vi "Tool measurment data collection.vi"(1 "Quer loop":u16, 2 "Stat 2 reader ID":i32, 11 "error out":errorcluster) -> ()   [LabVIEW 2011]
uses:
  LEINmaster/Defenitions/LEIN Structure variations.ctl
  LEINmaster/Defenitions/LEIN CMD List.ctl
  Stroker/Stat def/Stroker system stat2.ctl
  LEINmaster/Nodes/Controller local stat2.ctl
  LEINmaster/Nodes/pressure stat2.ctl
  LEINmaster/Nodes/solonoid stat2.ctl
  LEINmaster/Nodes/PSU stat2.ctl
  LEINmaster/Nodes/tensionsub stat2.ctl
  LEINmaster/Nodes/STAT2 data carrier type aware.ctl
  List of tools.ctl
  emi Lib/System 01/0 - General/App/Loop control 2/Private/_emi_ SMLoop start condition.vi
  emi Lib/System 01/0 - General/App/Loop control 2/Private/_emi_ SMLoop Error Check.vi
  emi Lib/Basic/0 - General/Error/emi_Is Error.vi
  emi Lib/System 01/0 - General/App/Loop control 2/Private/_emi_SMLoop Register new.vi
  emi Lib/System 01/0 - General/S&E reporting/emi_Send S&E Error message.vi
  emi Lib/Basic/0 - General/Error/emi_ Is Error state.vi
  emi Lib/System 01/0 - General/emi_Read System ID.vi
  emi Lib/System 01/0 - General/App/Loop control/Private/_emi_GFV Loop Linking.vi
  emi Lib/System 01/0 - General/App/Loop control/Private/_emi_GFV Loop Enable.vi
  emi Lib/System 01/0 - General/App/Loop control 2/Private/_emi_ SMLoop Restart.vi
  emi Lib/System 01/0 - General/App/Private/_emi_GFV App Close.vi
  emi Lib/System 01/0 - General/App/Loop control 2/Private/_emi_ SMLoop Restart Counter.vi
  emi Lib/System 01/0 - General/App/Loop control/Private/_emi_GFV Loop Running.vi
  emi Lib/System 01/0 - General/Private/_emi_GFV System ID.vi
  emi Lib/System 01/0 - General/S&E reporting/Private/_emi_S&E Q Generator.vi
  <vilib>/Utility/error.llb/Clear Errors.vi
  emi Lib/System 01/0 - General/App/Loop control/Private/_emi_GFV stop a loop so it can reset.vi
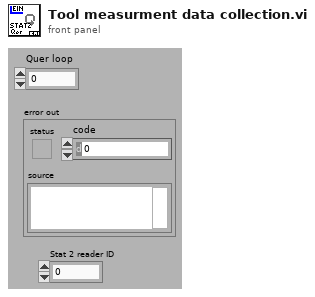
[diagram p1: front panel]
types:
  T1 = typedef "LEIN custom reply Q.ctl" = refnum<queue>
  T2 = typedef "LEIN CMD List.ctl" = enum8{"ACTI", "TASK", "RES0", "STAT", "RES1", "RES2", "RES3", "USER"}
  T3 = typedef "Stroker system stat2.ctl" = cluster{"Controller local":T4, "pressure 1":T5, "pressure 2":T5, "solonoid":T6, "PSU":T7, "Tension Sub 1":T8, "Tension Sub 2":T8}
  T4 = typedef "Controller local stat2.ctl" = cluster{"sys register":u16, "temperature":u16, "Input voltage":u16, "Input Current":u16, "Accelerometer ch0":u16, "Accelerometer ch1":u16, "Accelerometer ch2":u16, "Relay status":u8, "GPIO values":u8, "Sensor 1":i32, "Sensor 2":i32, "NA":u8, "High G monitoring":u8}
  T5 = typedef "pressure stat2.ctl" = cluster{"sys register":u16, "temperature":u16, "Pressure":u16, "osctun":u8}
  T6 = typedef "solonoid stat2.ctl" = cluster{"sys register":u16, "temperature":u16, "Position":i16, "monitor state":u8, "valve status":u8}
  T7 = typedef "PSU stat2.ctl" = cluster{"sys register":u16, "temperature":u16, "HV Voltage in":u16, "Main Voltage out":u16, "Main Current out":u16}
  T8 = typedef "tensionsub stat2.ctl" = cluster{"sys register":u16, "temperature":u16, "Tension":i16, "osctun":u8}
  T9 = typedef "STAT2 data carrier type aware.ctl" = cluster{"Tool":T10, "Data":variant}
  T10 = typedef "List of tools.ctl" = enum16{"Stroker", "Driller", "Tractor"}
  T11 = enum16{"big-endian, network order", "native, host order", "little-endian"}
  T12 = typedef "_emi_ SMLoop sates.ctl" = enum16{"Init", "Standby", "Start", "Normal Operation", "Stop", "Error Handling", "End", "Post"}
  T13 = cluster{"Placeholder":bool, "time valid receive":i32}
  T14 = typedef "LEIN Reply Holder.ctl" = cluster{"Reply msg(cmdif no reply)":T15, "Reply time":timestamp, "Valid reply":bool}
  T15 = typedef "LEIN CMD Cluster.ctl" = cluster{"SID":u8, "ANF":bool, "CMD":T2, "DATA":u8[]}
  T16 = typedef "LEIN Structure variations.ctl" = enum16{"LEIN08", "LEIN31", "LEIN63"}
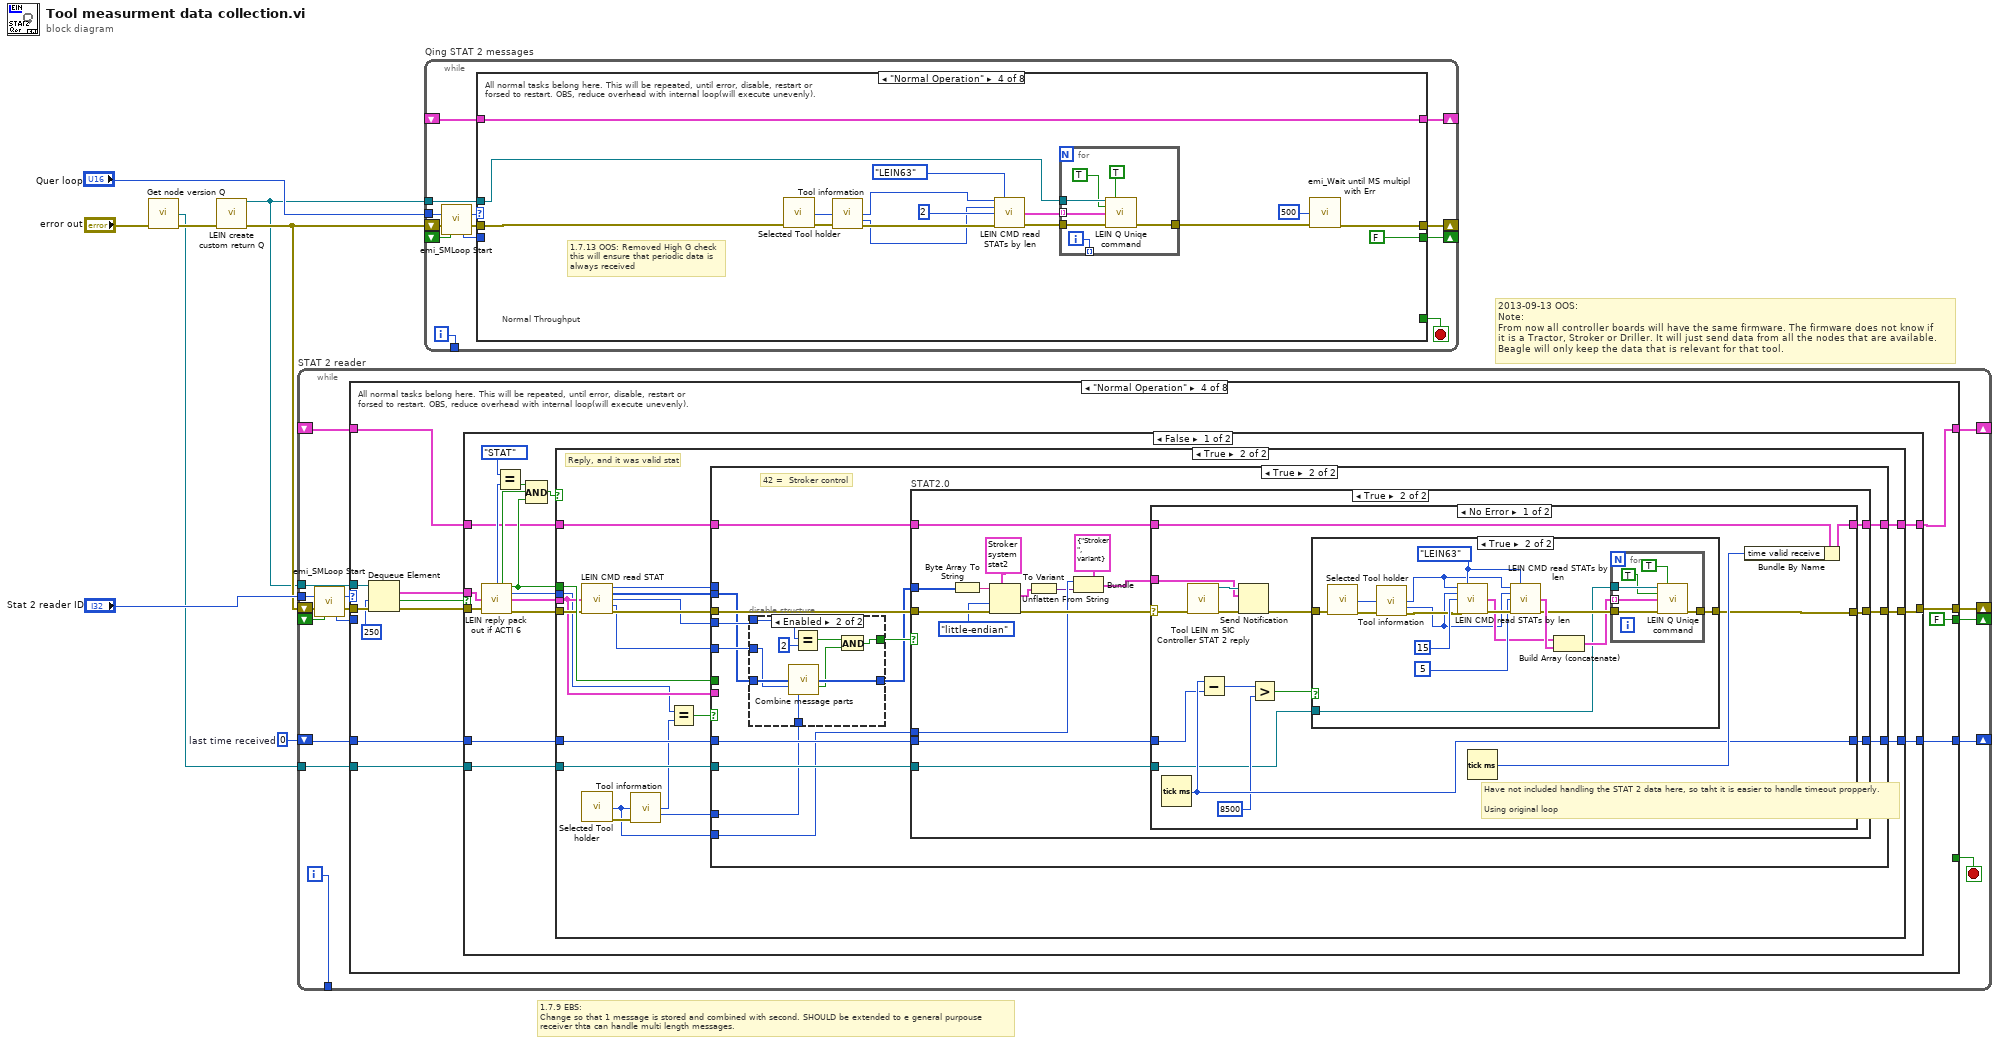
[diagram p0: block diagram]
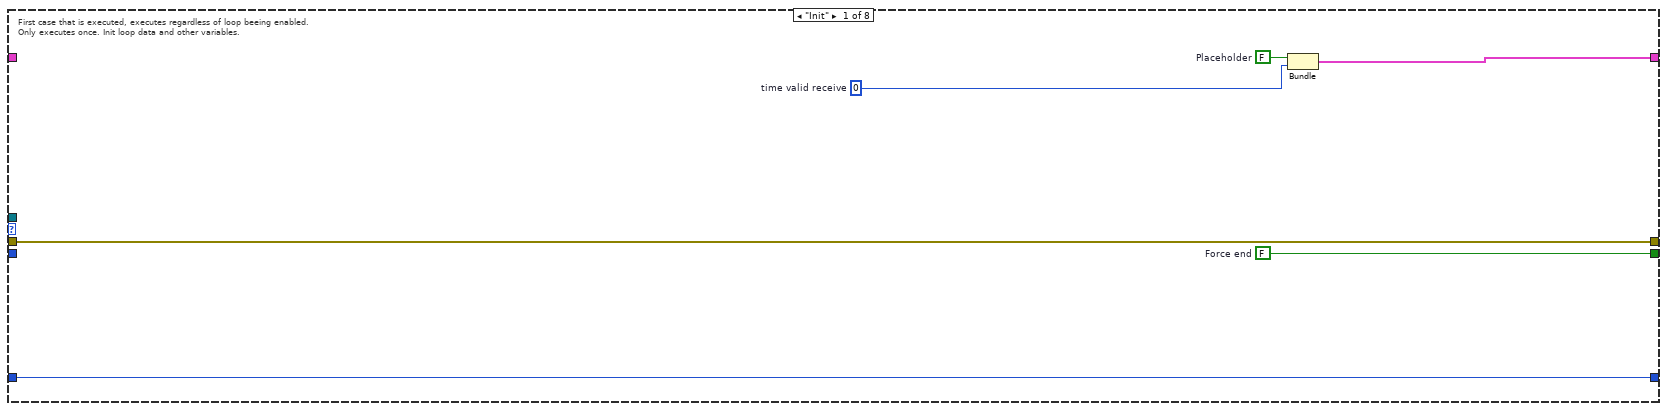
[diagram p2: hidden frame]
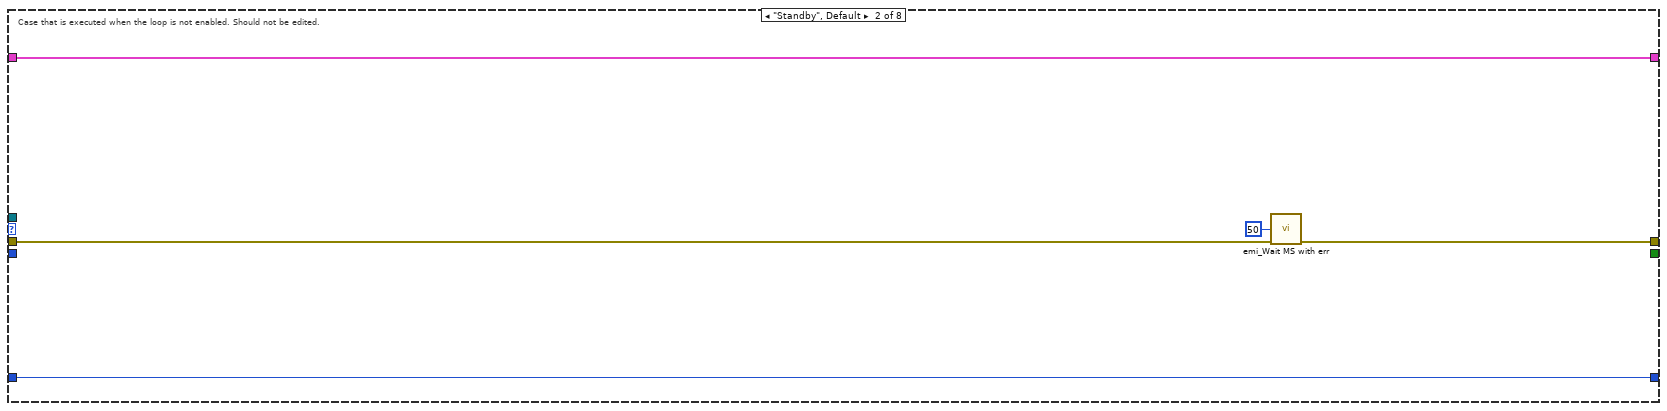
[diagram p3: hidden frame]
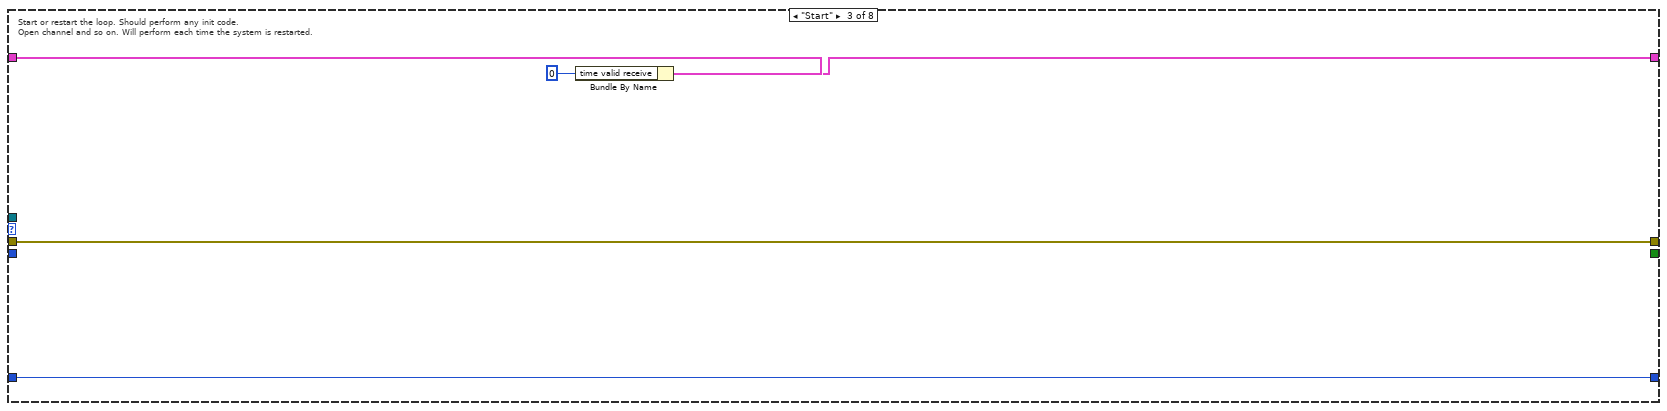
[diagram p4: hidden frame]
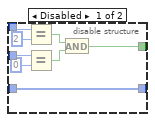
[diagram p7: hidden frame]
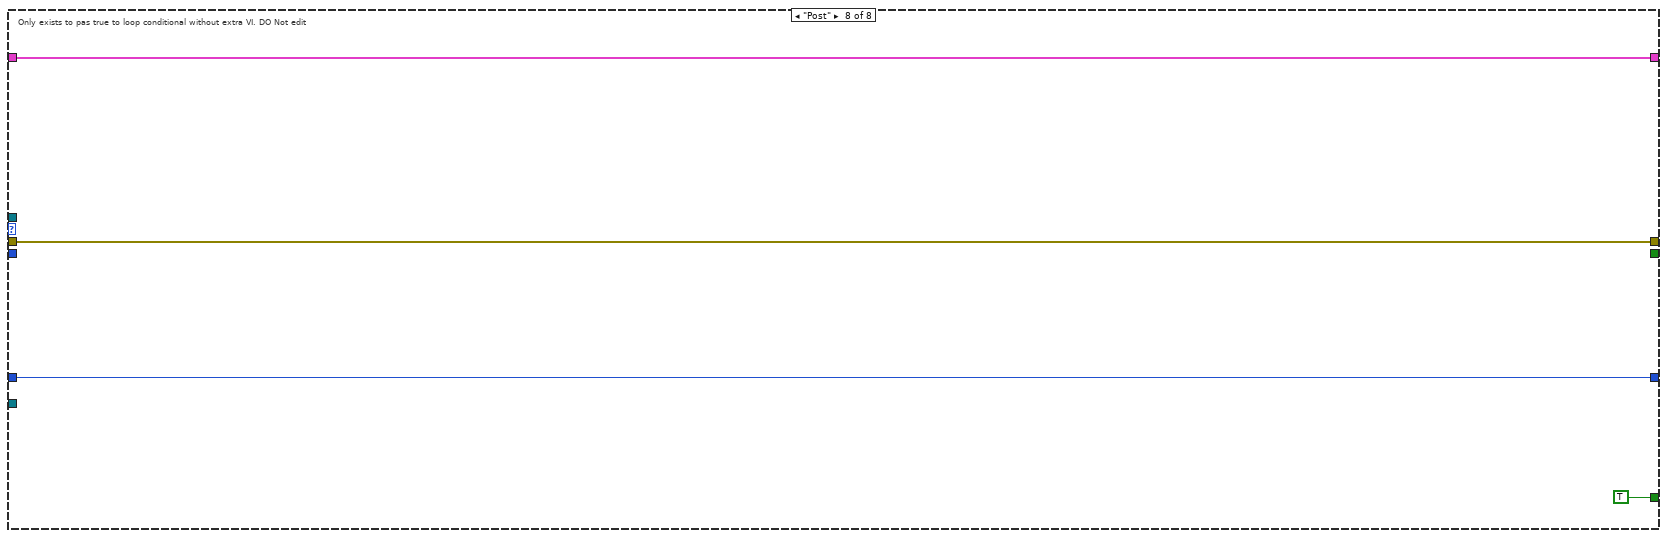
[diagram p15: hidden frame]
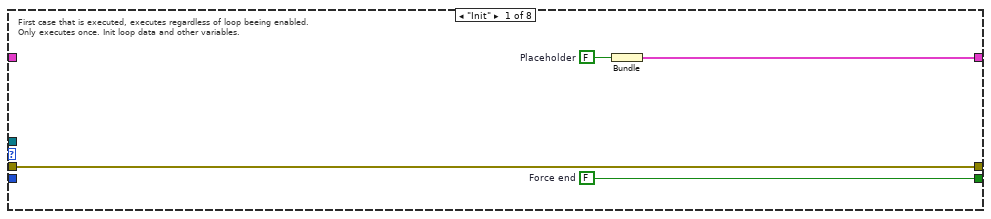
[diagram p16: hidden frame]
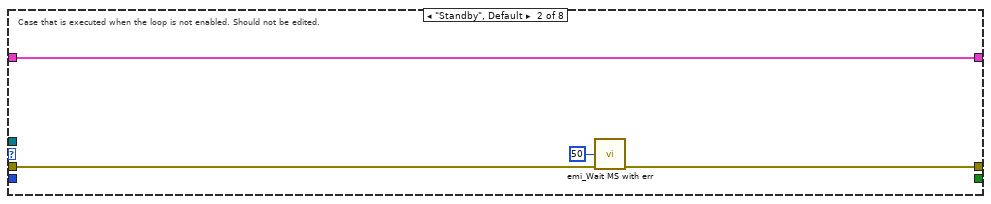
[diagram p17: hidden frame]
diagram:
  w4 = u32 0  # last time received
  # "2013-09-13 OOS:\nNote: \nFrom now all controller boards will have the same firmware. The firmware does not know if\nit is a Tractor, Stroker or Driller. It will just send data from all the nodes that are available. \nBeagle will only keep the data that is relevant for that tool."
  # "1.7.9 EBS:\nChange so that 1 message is stored and combined with second. SHOULD be extended to e general purpouse \nreceiver thta can handle multi length messages."
  n1 = call "Get node version Q.vi"("error in"="error out") -> ("LEIN custom reply Q"=w1:T1, "error out"=w2:errorcluster)  [unwired: 13 in]
  n2 = call "LEIN create custom return Q.vi"("error in (no error)"=w2) -> ("LEIN custom reply Q"=w5:T1, "error out"=w6:errorcluster)  [unwired: 13 in]
  n3 = while "STAT 2 reader" {
    shift-right: [w24] -> _
    shift-left: _ -> [w20]
    shift-right: [w22] -> _
    shift-left: w6 -> [w18]
    tunnel: [w21] -> _
    shift-right: [w19] -> _
    shift-left: _ -> [w14]
    tunnel: "Stat 2 reader ID" -> [w15]
    tunnel: w5 -> [w12]
    shift-right: [w11] -> _
    shift-left: w4 -> [w10]
    tunnel: w1 -> [w9]
    i -> [w21]
    stop <- w23 stop-if-true
    n4 = call "emi_SMLoop Start.vi"("Loop ID"=w15, "error in (no error)"=w18, "Force Stop(F)"=w14) -> ("Loop command"=w16:T12, "error out"=w17:errorcluster, "Loop ID out"=w13:i32)  [unwired: 10 in]
    n5 = case shown="\"Normal Operation\"" w16 {
      tunnel: [w29 w32 w38 w44 w193 w197 w199 w203] -> w24
      tunnel: [_ _ _ _ _ _ _ TRUE] -> w23
      tunnel: w17 -> [w30 w34 w40 w52 w194 w196 w200 w204]
      tunnel: [w30 w33 w40 w47 w194 w196 w200 w204] -> w22
      tunnel: w20 -> [_ w32 w39 w45 w193 w197 w199 w203]
      tunnel: [w27 _ _ FALSE ("Force End") _ _ _ _] -> w19
      tunnel: w13 -> [_ _ _ _ _ _ _ _]
      tunnel: w12 -> [_ _ _ w51 _ _ _ _]
      tunnel: [w25 w31 w36 w43 w192 w195 w198 w201] -> w11
      tunnel: w10 -> [w25 w31 w36 w42 w192 w195 w198 w201]
      tunnel: w9 -> [_ _ _ w41 _ _ _ _]
      frame "Init" {
        w26 = 0  # time valid receive
        w27 = FALSE  # Force end
        w28 = FALSE  # Placeholder
        # "First case that is executed, executes regardless of loop beeing enabled.\nOnly executes once. Init loop data and other variables."
        n6 = Bundle("Placeholder"=w28, "time valid receive"=w26) -> (w29:T13)  [unwired: 1 in]
      }
      frame "Standby", Default {
        # "Case that is executed when the loop is not enabled. Should not be edited."
        n7 = call "emi_Wait MS with err.vi"("milliseconds to wait(0)"=u32 50, "error in (no error)"=w34) -> ("error out"=w33:errorcluster)  [unwired: 13 in]
      }
      frame "Start" {
        # "Start or restart the loop. Should perform any init code. \nOpen channel and so on. Will perform each time the system is restarted."
        n8 = Bundle By Name(cluster=w39, "time valid receive"=0) -> (w38:T13)
      }
      frame "Normal Operation" {
        # "All normal tasks belong here. This will be repeated, until error, disable, restart or\nforsed to restart. OBS, reduce overhead with internal loop(will execute unevenly)."
        n9 = Dequeue Element(queue=w51, timeout in ms (-1)=250, error in (no error)=w52) -> (element=w46:T14, timed out?=w49:bool, error out=w48:errorcluster)  [unwired: 1 out]
        n10 = case shown="False" w49 {
          tunnel: w48 -> [w70 w190]
          tunnel: [w67 w190] -> w47
          tunnel: w46 -> [w69 _]
          tunnel: w45 -> [w58 w191]
          tunnel: [w57 w191] -> w44
          tunnel: [w56 w189] -> w43
          tunnel: w42 -> [w55 w189]
          tunnel: w41 -> [w54 _]
          frame False {
            n11 = call "LEIN reply pack out if ACTI 6.vi"("LEIN reply holder"=w69, "error in (no error)"=w70) -> ("CMD"=w61:T2, "Valid reply"=w64:bool, "ANF"=w62:bool, "SID"=w65:u8, "Reply(CMD if no reply)"=w66:T15, "error out"=w68:errorcluster)  [unwired: 8 in]
            n12 = Equal?(x=LEIN_CMD_List."STAT", y=w61) -> (x = y?=w59:bool)
            n13 = Compound Arithmetic op=AND(w59, w64, w62) -> (w63:bool)
            n14 = case shown="True" w63 {
              tunnel: w68 -> [w73 w91]
              tunnel: [w73 w93] -> w67
              tunnel: w66 -> [_ w90]
              tunnel: w65 -> [_ w78]
              tunnel: w62 -> [_ w92]
              tunnel: w58 -> [w72 w84]
              tunnel: [w72 w83] -> w57
              tunnel: [w71 w82] -> w56
              tunnel: w55 -> [w71 w81]
              tunnel: w54 -> [_ w80]
              frame False {
                # "No reply, or a NACK reply."
              }
              frame True {
                # "Reply, and it was valid stat"
                n15 = call "LEIN CMD read STAT.vi"("CMD"=w90, "error in (no error)"=w91) -> ("SID"=w86:u8, "Data"=w88:u8[], "STAT ID"=w87:u8, "STAT Part"=w85:u8, "error out"=w89:errorcluster)  [unwired: 8 in, 1 out]
                n16 = call "Selected Tool holder.vi"() -> ("Tool out"=w75:T10, "error out"=w76:errorcluster)  [unwired: 14 in]
                n17 = call "Tool information.vi"("Tool in"=w75, "error in (no error)"=w76) -> ("Main node address"=w79:u8, "Expected stat 2 message len"=w74:u8)  [unwired: 10 in, 2 out]
                n18 = Equal?(x=w78, y=w79) -> (x = y?=w77:bool)
                n19 = case shown="True" w77 {
                  tunnel: [w96 w107] -> w93
                  tunnel: w89 -> [w96 w106]
                  tunnel: w90 -> [_ _]
                  tunnel: w92 -> [_ _]
                  tunnel: w88 -> [_ w100]
                  tunnel: w87 -> [_ w109]
                  tunnel: w86 -> [_ _]
                  tunnel: w85 -> [_ w110]
                  tunnel: w84 -> [w95 w105]
                  tunnel: [w95 w104] -> w83
                  tunnel: [w94 w103] -> w82
                  tunnel: w81 -> [w94 w102]
                  tunnel: w80 -> [_ w101]
                  tunnel: w75 -> [_ w97]
                  tunnel: w74 -> [_ w98]
                  frame False {
                    # "TODO: Error?"
                  }
                  frame True {
                    # "42 =  Stroker control"
                    n20 = disable-structure shown="Enabled" {
                      disable-tunnel: w110 -> [w118 w121]
                      disable-tunnel: w109 -> [w117 w127]
                      disable-tunnel: [w112 w124] -> w108
                      disable-tunnel: w100 -> [w111 w123]
                      disable-tunnel: [w111 w122] -> w99
                      disable-tunnel: w98 -> [_ w119]
                      frame Disabled {
                        n21 = Equal?(x=w117, y=u8 2) -> (x = y?=w114:bool)
                        n22 = Equal?(x=w118, y=u8 0) -> (x = y?=w113:bool)
                        n23 = And(x=w114, y=w113) -> (x .and. y?=w112:bool)
                      }
                      frame Enabled {
                        n24 = call "Combine message parts.vi"("Data"=w123, "part"=w121, "Expected bytes"=w119) -> ("Data complete"=w122:u8[], "Complete data"=w120:bool)  [unwired: 11 in]
                        n25 = Equal?(x=w127, y=u8 2) -> (x = y?=w125:bool)
                        n26 = And(x=w125, y=w120) -> (x .and. y?=w124:bool)
                      }
                    }
                    n27 = case "STAT2.0" shown="True" w108 {
                      tunnel: [w129 w142] -> w107
                      tunnel: w106 -> [w129 w147]
                      tunnel: w99 -> [_ w146]
                      tunnel: w105 -> [w130 w144]
                      tunnel: [w130 w143] -> w104
                      tunnel: [w128 w140] -> w103
                      tunnel: w102 -> [w128 w139]
                      tunnel: w101 -> [_ w138]
                      tunnel: w97 -> [_ w137]
                      frame False {
                      }
                      frame True {
                        n28 = Byte Array To String(unsigned byte array=w146) -> (string=w136:string)
                        n29 = Unflatten From String(type=T3 {"Controller local"={"sys register"=0, "temperature"=0, "Input voltage"=0, "Input Current"=0, "Accelerometer ch0"=0, "Accelerometer ch1"=0, "Accelerometer ch2"=0, "Relay status"=0, "GPIO values"=0, "Sensor 1"=0, "Sensor 2"=0, "NA"=0, "High G monitoring"=0}, "pressure 1"={"sys register"=0, "temperature"=0, "Pressure"=0, "osctun"=0}, "pressure 2"={"sys register"=0, "temperature"=0, "Pressure"=0, "osctun"=0}, "solonoid"={"sys register"=0, "temperature"=0, "Position"=0, "monitor state"=0, "valve status"=0}, "PSU"={"sys register"=0, "temperature"=0, "HV Voltage in"=0, "Main Voltage out"=0, "Main Current out"=0}, "Tension Sub 1"={"sys register"=0, "temperature"=0, "Tension"=0, "osctun"=0}, "Tension Sub 2"={"sys register"=0, "temperature"=0, "Tension"=0, "osctun"=0}} ("system stat2"), binary string=w136, byte order (0:big-endian, network order)=T11."little-endian", error in (no error)=w147) -> (value=w132:T3, error out=w145:errorcluster)  [unwired: 1 in, 1 out]
                        n30 = To Variant(anything=w132) -> (Variant=w131:variant)
                        n31 = Bundle(cluster=T9 {"Tool"=enum."Stroker", "Data"=variant}, "Tool"=w137, "Data"=w131) -> (w141:T9)
                        n32 = case shown="No Error" w145 {
                          selector: w145 -> [w158 w187]
                          tunnel: w144 -> [w162 w188]
                          tunnel: [w161 w188] -> w143
                          tunnel: [w151 w187] -> w142
                          tunnel: w141 -> [w156 _]
                          tunnel: [w155 w186] -> w140
                          tunnel: w139 -> [w154 w186]
                          tunnel: w138 -> [w149 _]
                          frame No Error {
                            # "Have not included handling the STAT 2 data here, so taht it is easier to handle timeout propperly.\n\nUsing original loop"
                            n33 = Tick Count (ms)() -> (millisecond timer value=w155:u32)
                            n34 = call "Tool LEIN m SIC Controller STAT 2 reply.vi"("error in (no error)"=w158) -> ("notifier out"=w159:refnum<notifier>, "error out"=w157:errorcluster)  [unwired: 13 in]
                            n35 = Subtract(x=w155, y=w154) -> (x-y=w153:u32)
                            n36 = Send Notification(notification=w156, notifier=w159, error in (no error)=w157) -> (error out=w148:errorcluster)  [unwired: 1 out]
                            n37 = Greater?(x=w153, y=u32 8500) -> (0:w150:bool)
                            n38 = case shown="True" w150 {
                              tunnel: [w163 w173] -> w151
                              tunnel: w148 -> [w163 w164]
                              tunnel: w149 -> [_ w170]
                              frame False {
                              }
                              frame True {
                                w176 = LEIN_Structure_variations."LEIN63" ("LEIN Variation")
                                n39 = call "Selected Tool holder.vi"("error in (no error)"=w164) -> ("Tool out"=w168:T10, "error out"=w169:errorcluster)  [unwired: 13 in]
                                n40 = call "Tool information.vi"("Tool in"=w168, "error in (no error)"=w169) -> ("Main node address"=w166:u8, "Expected stat 2 message len"=w165:u8, "error out"=w167:errorcluster)  [unwired: 10 in, 1 out]
                                n41 = call "LEIN CMD read STATs by len.vi"("SID"=w166, "LEIN Variation"=w176, "Expected LEN"=w165, "STAT ID"=u8 15, "error in"=w167) -> ("STATs"=w174:T15[], "error out"=w178:errorcluster)  [unwired: 9 in]
                                n42 = call "LEIN CMD read STATs by len.vi"("SID"=w166, "LEIN Variation"=w176, "Expected LEN"=w165, "STAT ID"=u8 5, "error in"=w178) -> ("STATs"=w175:T15[], "error out"=w172:errorcluster)  [unwired: 9 in]
                                n43 = Build Array (concatenate)(w174, w175) -> (w171:T15[])
                                n44 = for {
                                tunnel: [w185] -> w173
                                tunnel: w172 -> [w184]
                                tunnel: w171 -> [w183] mode=indexing
                                tunnel: w170 -> [w181]
                                n45 = call "LEIN Q Uniqe command.vi"("LEIN custom reply Q"=w181, "Retry on err (F)"=TRUE, "Custom Q(F)"=TRUE, "CMD"=w183, "error in"=w184) -> ("error out"=w185:errorcluster)  [unwired: 10 in]
                                }
                              }
                            }
                            n46 = Tick Count (ms)() -> (millisecond timer value=w160:u32)
                            n47 = Bundle By Name(cluster=w162, "time valid receive"=w160) -> (w161:T13)
                          }
                          frame Error {
                          }
                        }
                      }
                    }
                  }
                }
              }
            }
          }
          frame True {
          }
        }
      }
      frame "Stop" {
        # "Stop the loop. May be restarted later. Close interfaces and the like"
      }
      frame "Error Handling" {
        # "Loop automaticaly returns here after error is found. If error is cleared, \nLoop wil continue as normal(if was operative when error."
      }
      frame "End" {
        # "Only executes at application end has. Should performa any action the loop \nneeds to finnish. Executes only once."
      }
      frame "Post" {
        # "Only exists to pas true to loop conditional without extra VI. DO Not edit"
      }
    }
  }
  n48 = while "Qing STAT 2 messages" {
    shift-right: [w217] -> _
    shift-left: _ -> [w213]
    shift-right: [w215] -> _
    shift-left: w6 -> [w211]
    tunnel: [w214] -> _
    shift-right: [w212] -> _
    shift-left: _ -> [w207]
    tunnel: "Quer loop" -> [w208]
    tunnel: w5 -> [w205]
    i -> [w214]
    stop <- w216 stop-if-true
    n49 = call "emi_SMLoop Start.vi"("Loop ID"=w208, "error in (no error)"=w211, "Force Stop(F)"=w207) -> ("Loop command"=w209:T12, "error out"=w210:errorcluster, "Loop ID out"=w206:i32)  [unwired: 10 in]
    n50 = case shown="\"Normal Operation\"" w209 {
      tunnel: [w220 w222 w226 w241 w251 w254 w255 w258] -> w217
      tunnel: [_ _ _ _ _ _ _ TRUE] -> w216
      tunnel: w210 -> [w221 w224 w227 w243 w252 w253 w256 w259]
      tunnel: [w221 w223 w227 w242 w252 w253 w256 w259] -> w215
      tunnel: w213 -> [_ w222 w226 w241 w251 w254 w255 w258]
      tunnel: [w218 _ _ FALSE ("Force End") _ _ _ _] -> w212
      tunnel: w206 -> [_ _ _ _ _ _ _ _]
      tunnel: w205 -> [_ _ _ w239 _ _ _ _]
      frame "Init" {
        w218 = FALSE  # Force end
        w219 = FALSE  # Placeholder
        # "First case that is executed, executes regardless of loop beeing enabled.\nOnly executes once. Init loop data and other variables."
        n51 = Bundle("Placeholder"=w219) -> (w220:cluster{"Placeholder":bool})  [unwired: 1 in]
      }
      frame "Standby", Default {
        # "Case that is executed when the loop is not enabled. Should not be edited."
        n52 = call "emi_Wait MS with err.vi"("milliseconds to wait(0)"=u32 50, "error in (no error)"=w224) -> ("error out"=w223:errorcluster)  [unwired: 13 in]
      }
      frame "Start" {
        # "Start or restart the loop. Should perform any init code. \nOpen channel and so on. Will perform each time the system is restarted."
      }
      frame "Normal Operation" {
        # "1.7.13 OOS: Removed High G check\nthis will ensure that periodic data is \nalways received"
        # "Normal Throughput"
        # "All normal tasks belong here. This will be repeated, until error, disable, restart or\nforsed to restart. OBS, reduce overhead with internal loop(will execute unevenly)."
        n53 = call "Selected Tool holder.vi"("error in (no error)"=w243) -> ("Tool out"=w231:T10, "error out"=w232:errorcluster)  [unwired: 13 in]
        n54 = call "Tool information.vi"("Tool in"=w231, "error in (no error)"=w232) -> ("Main node address"=w230:u8, "Expected stat 2 message len"=w228:u8, "error out"=w229:errorcluster)  [unwired: 10 in, 1 out]
        n55 = call "LEIN CMD read STATs by len.vi"("SID"=w230, "LEIN Variation"=LEIN_Structure_variations."LEIN63", "Expected LEN"=w228, "STAT ID"=u8 2, "error in"=w229) -> ("STATs"=w234:T15[], "error out"=w235:errorcluster)  [unwired: 9 in]
        n56 = for {
          tunnel: [w250] -> w237
          tunnel: w235 -> [w249]
          tunnel: w234 -> [w248] mode=indexing
          tunnel: w239 -> [w246]
          tunnel: [w244] -> _ mode=indexing
          i -> [w244]
          n57 = call "LEIN Q Uniqe command.vi"("LEIN custom reply Q"=w246, "Retry on err (F)"=TRUE, "Custom Q(F)"=TRUE, "CMD"=w248, "error in"=w249) -> ("error out"=w250:errorcluster)  [unwired: 10 in]
        }
        n58 = call "emi_Wait until MS multipl with Err.vi"("millisecond multiple(0)"=u32 500 ("milliseconds to wait(0)"), "error in (no error)"=w237) -> ("error out"=w242:errorcluster)  [unwired: 13 in]
      }
      frame "Stop" {
        # "Stop the loop. May be restarted later. Close interfaces and the like"
      }
      frame "Error Handling" {
        # "Loop automaticaly returns here after error is found. If error is cleared, \nLoop wil continue as normal(if was operative when error."
      }
      frame "End" {
        # "Only executes at application end has. Should performa any action the loop \nneeds to finnish. Executes only once."
      }
      frame "Post" {
        # "Only exists to pas true to loop conditional without extra VI. DO Not edit"
      }
    }
  }
